vi "LS4 GetPosSingleAxis_SD.vi"(0 "Axis":i32=1) -> (1 "Command executed":bool, 2 "Pos":dbl format="%.3f")   [LabVIEW 2015]
doc: "This VI returns the position of a single axis (1..4)."
uses:
  DLL/LStep4.dll
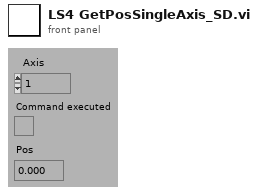
[diagram p1: front panel]
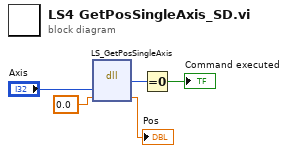
[diagram p0: block diagram]
diagram:
  n1 = dll-call lib="G:/SD/TRANCON-2015/DLL/LStep4.dll" fn="LS_GetPosSingleAxis"("Axis"="Axis", "Pos"=0.0) -> ("type de retour"=w5:i32, "Pos"=→"Pos":dbl)  [unwired: 4 in, 2 out]
  n2 = Equal To 0?(x=w5) -> (x = 0?=→"Command executed":bool)
